vi "Request ID.vi"(11 "IErrorHandler in":refnum<class "IErrorHandler.lvclass">) -> (2 "Request ID":u64, 3 "IErrorHandler out":refnum<class "IErrorHandler.lvclass">)   [LabVIEW 2020, in "wamplv.lvlib" / "IErrorHandler.lvclass"]
uses:
  IErrorHandler.lvclass
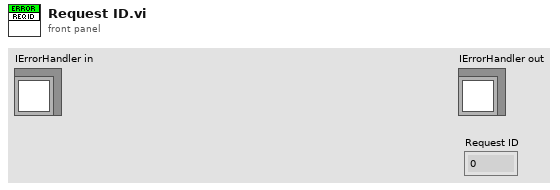
[diagram p1: front panel]
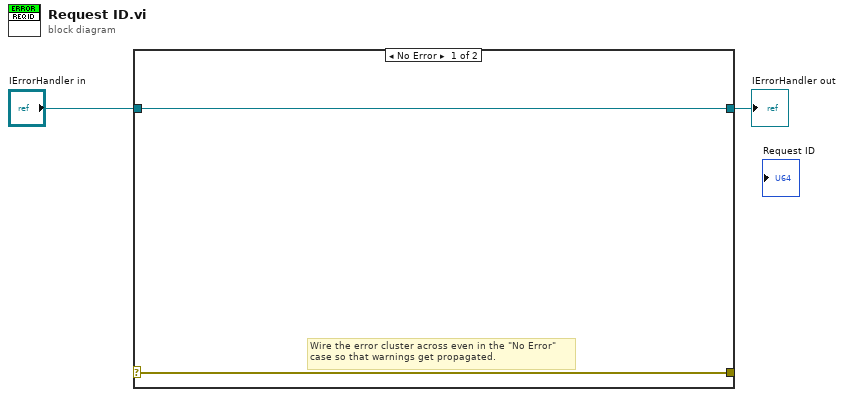
[diagram p0: block diagram]
diagram:
  n1 = case shown="No Error" {
    selector: _ -> [w3 w6]
    tunnel: [w3 w6] -> _
    tunnel: [w4 w5] -> w1
    tunnel: "IErrorHandler in" -> [w4 w5]
    frame No Error {
      # "Wire the error cluster across even in the \"No Error\"\ncase so that warnings get propagated."
    }
    frame Error {
    }
  }
  "IErrorHandler out" <- w1
